vi "DiffDriveVoltageConstraint_getMinMaxAccel.vi"(8 "Velocity":dbl, 9 "Curvature":dbl, 10 "statePose":T5={"TRANSLATION"={"X"=0.0, "Y"=0.0}, "ROTATION"={"VALUE"=0.0, "COS"=1.0, "SIN"=0.0}} {"ROTATION"."SIN" format="%13.4f"; "ROTATION"."COS" format="%13.4f"; "ROTATION"."VALUE" format="%13.4f"; "TRANSLATION"."Y" format="%14.3f"; "TRANSLATION"."X" format="%14.3f"}, 11 "DIFF_DRIVE_VOLTAGE_CONSTRAINT":T1 {"SIMPLE_MOTOR_FF"."Ka" format="%13.4f"; "SIMPLE_MOTOR_FF"."Kv" format="%13.4f"; "SIMPLE_MOTOR_FF"."Ks" format="%13.4f"; "DIFF_DRIVE_KINEMATICS"."TrackWidth_Meters" format="%20.4f"; "Max Voltage" format="%20.4f"}) -> (3 "TRAJ_CONSTAINT_MIN_MAX":T4)   [LabVIEW 2019, in "Trajectory_Library.lvlib"]
doc: "Return the minimum and maximum allowed acceleration given the provided conditions.\n\nIt appears that this routine doesn't do anything. It returns default values.\n\nParameters:\n - DiffDriveVoltageConstraint - Constraint data structure\n - statePose - current traj state Pose\n - curvature - current traj curvature\n - maxVelocity - current traj max velocity\n\nReturns\n - TrajConstraint_Min_Max - Data structure with Min / Max acceleration."
uses:
  Trajectory_Library.lvlib
  TypeDef/POSE2D.ctl
  TypeDef/TRANSLATION2D.ctl
  TypeDef/ROTATION2D.ctl
  TypeDef/TRAJ_CONSTRAINT_MINMAX.ctl
  TypeDef/TRAJ_CONSTRAINT_DIIF_DRIVE_VOLTAGE.ctl
  TypeDef/DIFF_DRIVE_KINEMATICS.ctl
  TypeDef/SIMPLE_MOTOR_FF.ctl
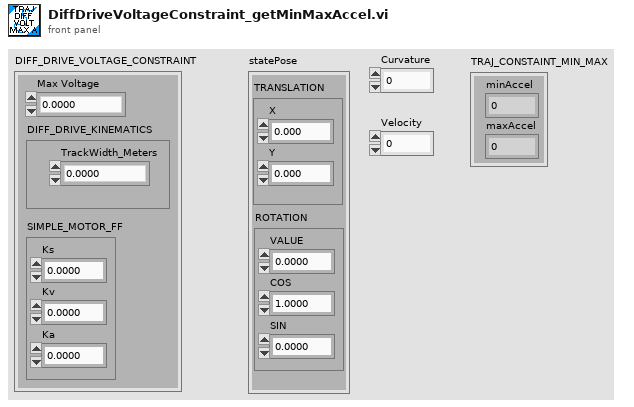
[diagram p1: front panel]
types:
  T1 = typedef "Trajectory_Library.lvlib/TRAJ_CONSTRAINT_DIIF_DRIVE_VOLTAGE.ctl" = cluster{"Max Voltage":dbl, "DIFF_DRIVE_KINEMATICS":T2, "SIMPLE_MOTOR_FF":T3}
  T2 = typedef "Trajectory_Library.lvlib/DIFF_DRIVE_KINEMATICS.ctl" = cluster{"TrackWidth_Meters":dbl}
  T3 = typedef "Trajectory_Library.lvlib/SIMPLE_MOTOR_FF.ctl" = cluster{"Ks":dbl, "Kv":dbl, "Ka":dbl}
  T4 = typedef "Trajectory_Library.lvlib/TRAJ_CONSTRAINT_MINMAX.ctl" = cluster{"minAccel":dbl, "maxAccel":dbl}
  T5 = typedef "Trajectory_Library.lvlib/POSE2D.ctl" = cluster{"TRANSLATION":T6, "ROTATION":T7}
  T6 = typedef "Trajectory_Library.lvlib/TRANSLATION2D.ctl" = cluster{"X":dbl, "Y":dbl}
  T7 = typedef "Trajectory_Library.lvlib/ROTATION2D.ctl" = cluster{"VALUE":dbl, "COS":dbl, "SIN":dbl}
  T8 = typedef "Trajectory_Library.lvlib/CHASSIS_SPEEDS.ctl" = cluster{"vX":dbl, "vY":dbl, "vOmega":dbl}
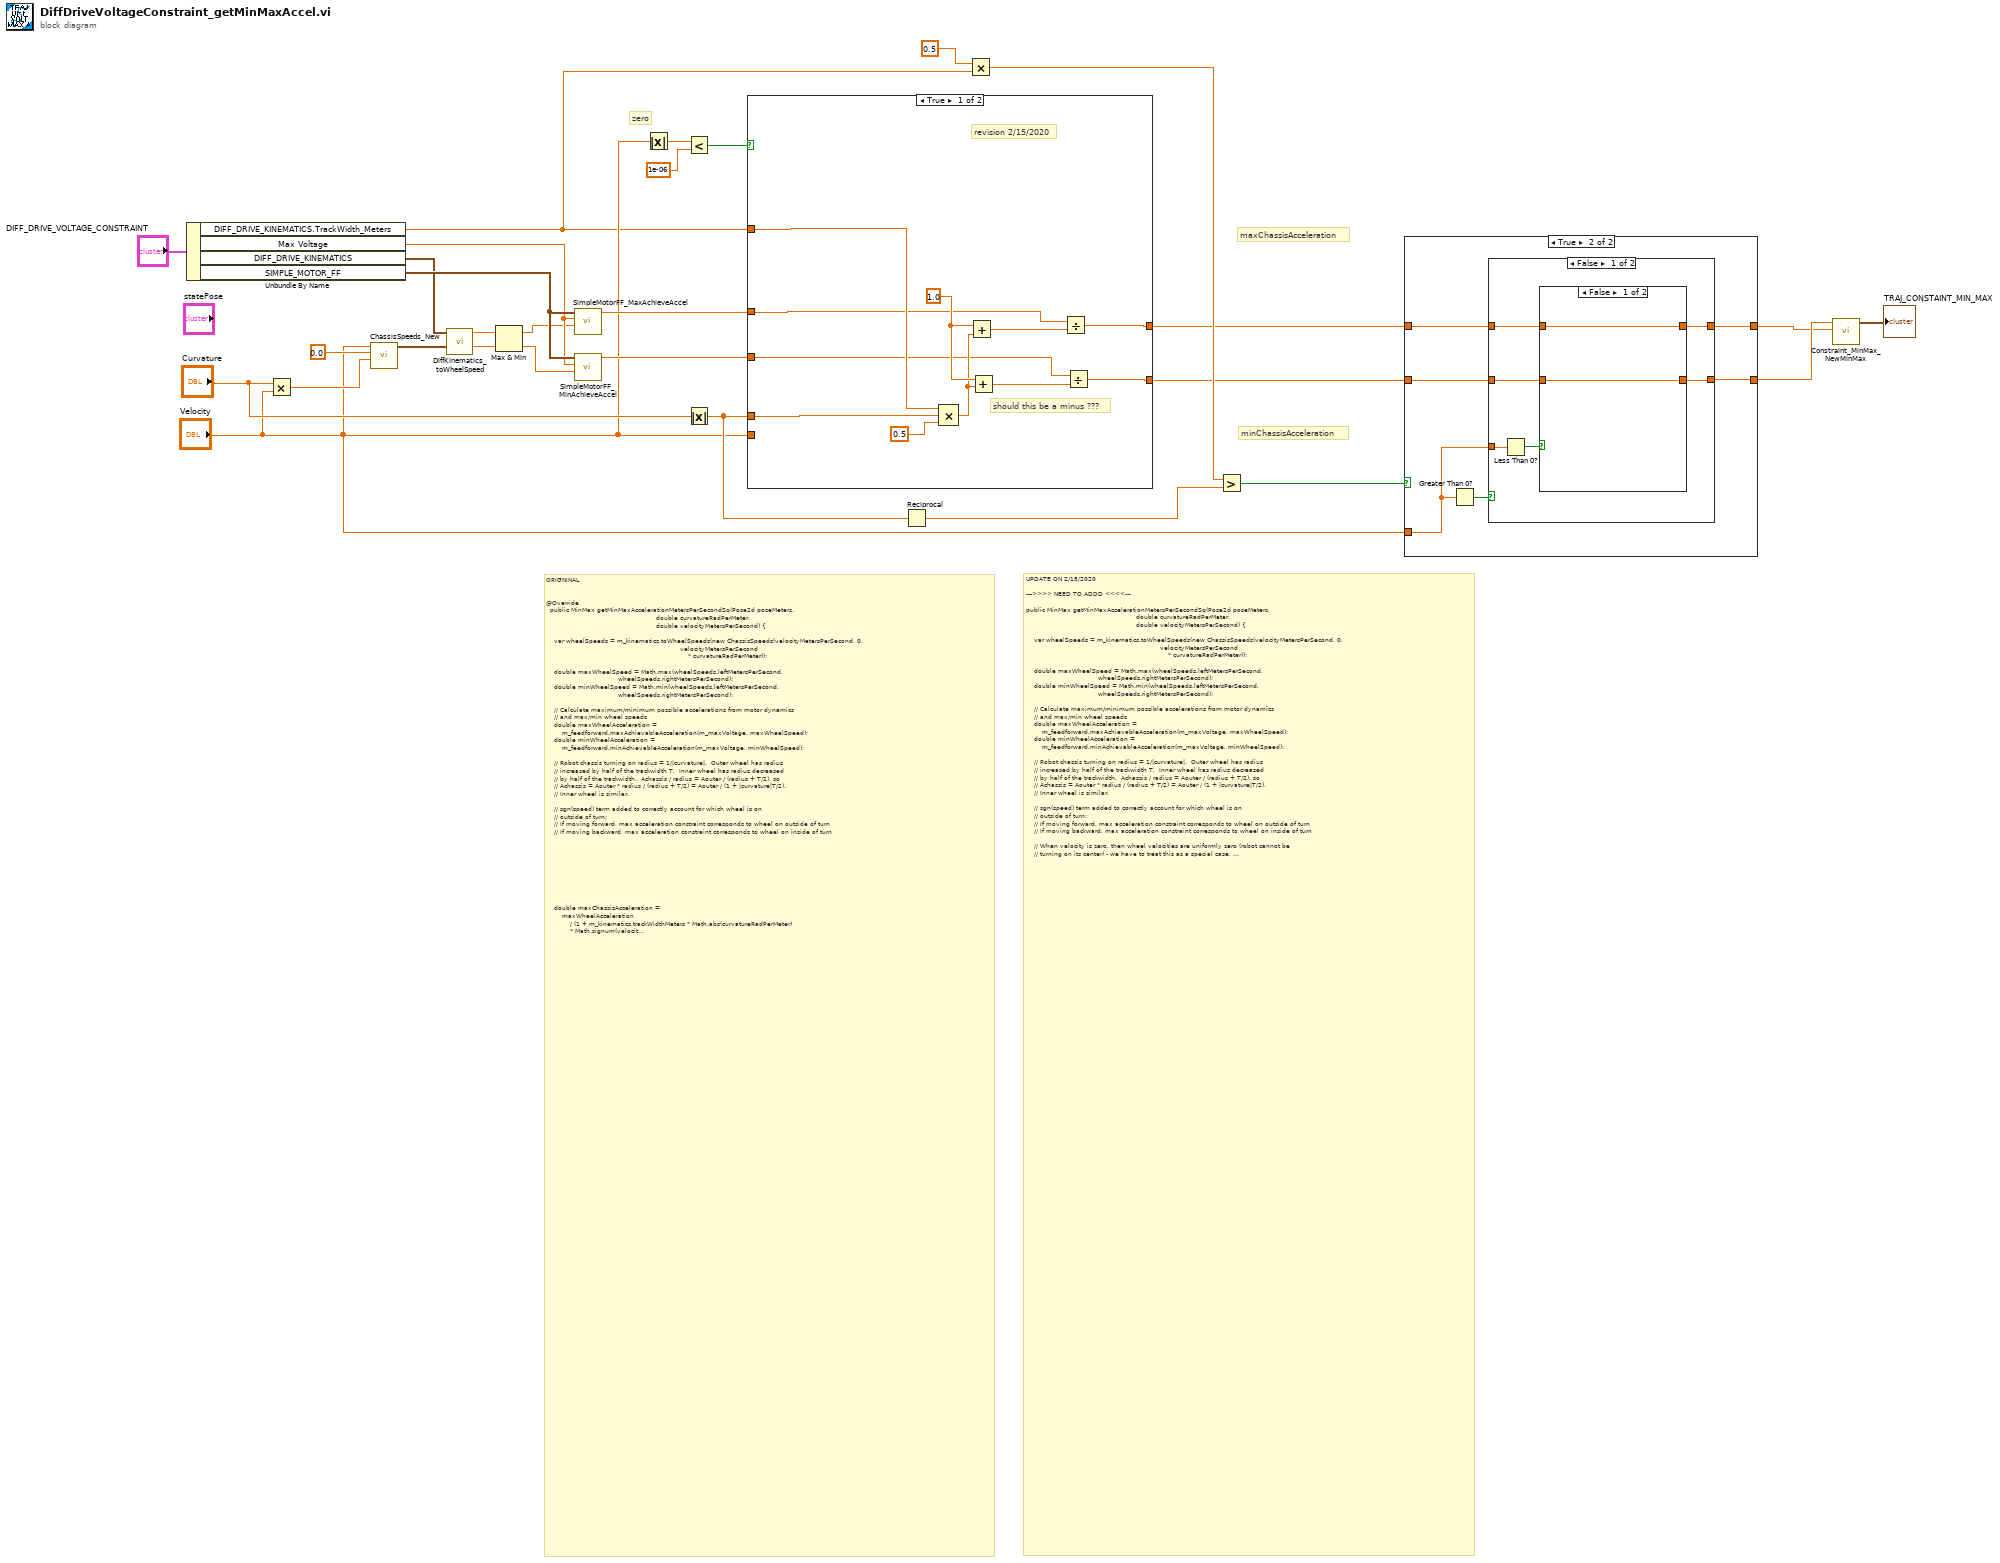
[diagram p0: block diagram]
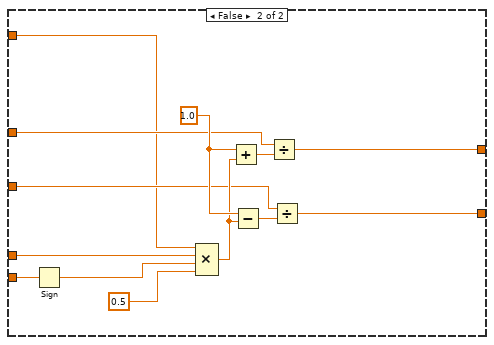
[diagram p2: hidden frame]
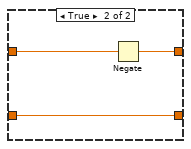
[diagram p4: hidden frame]
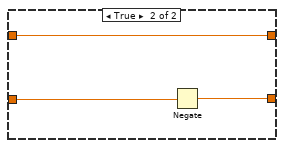
[diagram p5: hidden frame]
diagram:
  # "minChassisAcceleration"
  # "maxChassisAcceleration"
  # "zero"
  # "UPDATE ON 2/15/2020\n\n--->>>> NEED TO ADDD <<<<---\n\npublic MinMax getMinMaxAccelerationMetersPerSecondSq(Pose2d poseMeters,\n                                                       double curvatureRadPerMeter,\n                                                       double velocityMetersPerSecond) {\n\n    var wheelSpeeds = m_kinematics.toWheelSpeeds(new ChassisSpeeds(velocityMetersPerSecond, 0,\n                                                                   velocityMetersPerSecond\n                                                                       * curvatureRadPerMeter));\n\n    double maxWheelSpeed = Math.max(wheelSpeeds.leftMetersPerSecond,\n                                    wheelSpeeds.rightMetersPerSecond);\n    double minWheelSpeed = Math.min(wheelSpeeds.leftMetersPerSecond,\n                                    wheelSpeeds.rightMetersPerSecond);\n\n    // Calculate maximum/minimum possible accelerations from motor dynamics\n    // and max/min wheel speeds\n    double maxWheelAcceleration =\n        m_feedforward.maxAchievableAcceleration(m_maxVoltage, maxWheelSpeed);\n    double minWheelAcceleration =\n        m_feedforward.minAchievableAcceleration(m_maxVoltage, minWheelSpeed);\n\n    // Robot chassis turning on radius = 1/|curvature|.  Outer wheel has radius\n    // increased by half of the trackwidth T.  Inner wheel has radius decreased\n    // by half of the trackwidth.  Achassis / radius = Aouter / (radius + T/2), so\n    // Achassis = Aouter * radius / (radius + T/2) = Aouter / (1 + |curvature|T/2).\n    // Inner wheel is similar.\n\n    // sgn(speed) term added to correctly account for which wheel is on\n    // outside of turn:\n    // If moving forward, max acceleration constraint corresponds to wheel on outside of turn\n    // If moving backward, max acceleration constraint corresponds to wheel on inside of turn\n\n    // When velocity is zero, then wheel velocities are uniformly zero (robot cannot be\n    // turning on its center) - we have to treat this as a special case, as it breaks\n    // the signum function.  Both max and min acceleration are *reduced in magnitude*\n    // in this case.\n\n    double maxChassisAcceleration;\n    double minChassisAcceleration;\n\n    if (velocityMetersPerSecond == 0) {\n      maxChassisAcceleration =\n          maxWheelAcceleration\n              / (1 + m_kinematics.trackWidthMeters * Math.abs(curvatureRadPerMeter) / 2);\n      minChassisAcceleration =\n          minWheelAcceleration\n              / (1 + m_kinematics.trackWidthMeters * Math.abs(curvatureRadPerMeter) / 2);\n    } else {\n      maxChassisAcceleration =\n          maxWheelAcceleration\n              / (1 + m_kinematics.trackWidthMeters * Math.abs(curvatureRadPerMeter)\n              * Math.signum(velocityMetersPerSecond) / 2);\n      minChassisAcceleration =\n          minWheelAcceleration\n              / (1 - m_kinematics.trackWidthMeters * Math.abs(curvatureRadPerMeter)\n              * Math.signum(velocityMetersPerSecond) / 2);\n    }\n\n    // When turning about a point inside of the wheelbase (i.e. radius less than half\n    // the trackwidth), the inner wheel's direction changes, but the magnitude remains\n    // the same.  The formula above changes sign for the inner wheel when this happens.\n    // We can accurately account for this by simply negating the inner wheel.\n\n    if ((m_kinematics.trackWidthMeters / 2) > (1 / Math.abs(curvatureRadPerMeter))) {\n      if (velocityMetersPerSecond > 0) {\n        minChassisAcceleration = -minChassisAcceleration;\n      } else if (velocityMetersPerSecond < 0) {\n        maxChassisAcceleration = -maxChassisAcceleration;\n      }\n    }\n\n    return new MinMax(minChassisAcceleration, maxChassisAcceleration);\n  }\n}"
  # "ORIGNINAL\n\n\n@Override\n  public MinMax getMinMaxAccelerationMetersPerSecondSq(Pose2d poseMeters,\n                                                       double curvatureRadPerMeter,\n                                                       double velocityMetersPerSecond) {\n\n    var wheelSpeeds = m_kinematics.toWheelSpeeds(new ChassisSpeeds(velocityMetersPerSecond, 0,\n                                                                   velocityMetersPerSecond\n                                                                       * curvatureRadPerMeter));\n\n    double maxWheelSpeed = Math.max(wheelSpeeds.leftMetersPerSecond,\n                                    wheelSpeeds.rightMetersPerSecond);\n    double minWheelSpeed = Math.min(wheelSpeeds.leftMetersPerSecond,\n                                    wheelSpeeds.rightMetersPerSecond);\n\n    // Calculate maximum/minimum possible accelerations from motor dynamics\n    // and max/min wheel speeds\n    double maxWheelAcceleration =\n        m_feedforward.maxAchievableAcceleration(m_maxVoltage, maxWheelSpeed);\n    double minWheelAcceleration =\n        m_feedforward.minAchievableAcceleration(m_maxVoltage, minWheelSpeed);\n\n    // Robot chassis turning on radius = 1/|curvature|.  Outer wheel has radius\n    // increased by half of the trackwidth T.  Inner wheel has radius decreased\n    // by half of the trackwidth.  Achassis / radius = Aouter / (radius + T/2), so\n    // Achassis = Aouter * radius / (radius + T/2) = Aouter / (1 + |curvature|T/2).\n    // Inner wheel is similar.\n\n    // sgn(speed) term added to correctly account for which wheel is on\n    // outside of turn:\n    // If moving forward, max acceleration constraint corresponds to wheel on outside of turn\n    // If moving backward, max acceleration constraint corresponds to wheel on inside of turn\n\n\n\n\n\n\n\n\n\n    double maxChassisAcceleration =\n        maxWheelAcceleration\n            / (1 + m_kinematics.trackWidthMeters * Math.abs(curvatureRadPerMeter)\n            * Math.signum(velocityMetersPerSecond) / 2);\n    double minChassisAcceleration =\n        minWheelAcceleration\n            / (1 - m_kinematics.trackWidthMeters * Math.abs(curvatureRadPerMeter)\n            * Math.signum(velocityMetersPerSecond) / 2);\n\n\n\n\n\n\n\n\n\n\n\n\n\n\n    // Negate acceleration of wheel on inside of turn if center of turn is inside of wheelbase\n    if ((m_kinematics.trackWidthMeters / 2) > (1 / Math.abs(curvatureRadPerMeter))) {\n      if (velocityMetersPerSecond > 0) {\n        minChassisAcceleration = -minChassisAcceleration;\n      } else {\n        maxChassisAcceleration = -maxChassisAcceleration;\n      }\n    }\n\n    return new MinMax(minChassisAcceleration, maxChassisAcceleration);\n  }"
  n1 = Unbundle By Name("DIFF_DRIVE_VOLTAGE_CONSTRAINT") -> ("DIFF_DRIVE_KINEMATICS.TrackWidth_Meters"=w2:dbl, "Max Voltage"=w27:dbl, "DIFF_DRIVE_KINEMATICS"=w26:T2, "SIMPLE_MOTOR_FF"=w28:T3)
  n2 = Multiply(x="Curvature", y="Velocity") -> (x*y=w24:dbl)
  n3 = call "ChassisSpeeds_New.vi"("vAngular"=w24, "vY"=0.0 ("vAngular"), "vX"="Velocity") -> ("CHASSIS"=w23:T8)  [unwired: 8 in]
  n4 = call "DiffKinematics_toWheelSpeed.vi"("CHASSIS Speed"=w23, "DIFF_DRIVE_KINEMATICS"=w26) -> ("RightVelocity"=w22:dbl, "LeftVelocity"=w21:dbl)  [unwired: 8 in]
  n5 = Max & Min(x=w21, y=w22) -> (max(x,y)=w20:dbl, min(x,y)=w19:dbl)
  n6 = call "SimpleMotorFF_MaxAchieveAccel.vi"("Velocity"=w20, "MaxVoltage"=w27, "SIMPLE_MOTOR_FF"=w28) -> ("MaxAccel"=w17:dbl)  [unwired: 8 in]
  n7 = call "SimpleMotorFF_MinAchieveAccel.vi"("Velocity"=w19, "MaxVoltage"=w27, "SIMPLE_MOTOR_FF"=w28) -> ("MinAccel"=w16:dbl)  [unwired: 8 in]
  n8 = Absolute Value(x="Velocity") -> (abs(x)=w5:dbl)
  n9 = Less?(x=w5, y=1e-06) -> (x < y?=w1:bool)
  n10 = Absolute Value(x="Curvature") -> (abs(x)=w12:dbl)
  n11 = case shown="True" w1 {
    tunnel: w17 -> [w33 w47]
    tunnel: w16 -> [w32 w46]
    tunnel: w12 -> [w31 w45]
    tunnel: [w36 w44] -> w10
    tunnel: [w35 w43] -> w9
    tunnel: "Velocity" -> [_ w42]
    tunnel: w2 -> [w34 w41]
    frame True {
      w40 = 1.0 ("x")
      # "revision 2/15/2020"
      # "should this be a minus ???"
      n12 = Compound Arithmetic op=MULTIPLY(w34, w31, 0.5 ("value")) -> (w39:dbl)
      n13 = Add(x=w40, y=w39) -> (x+y=w38:dbl)
      n14 = Add(x=w40, y=w39) -> (x+y=w37:dbl)
      n15 = Divide(x=w33, y=w38) -> (x/y=w36:dbl)
      n16 = Divide(x=w32, y=w37) -> (x/y=w35:dbl)
    }
    frame False {
      w51 = 1.0 ("x")
      n17 = Sign(1:w42) -> (0:w53:dbl)
      n18 = Compound Arithmetic op=MULTIPLY(w41, w45, w53, 0.5 ("value")) -> (w50:dbl)
      n19 = Add(x=w51, y=w50) -> (x+y=w49:dbl)
      n20 = Subtract(x=w51, y=w50) -> (x-y=w48:dbl)
      n21 = Divide(x=w47, y=w49) -> (x/y=w44:dbl)
      n22 = Divide(x=w46, y=w48) -> (x/y=w43:dbl)
    }
  }
  n23 = Reciprocal(x=w12) -> (1/x=w11:dbl)
  n24 = Multiply(x=0.5, y=w2) -> (x*y=w13:dbl)
  n25 = Greater?(x=w13, y=w11) -> (0:w14:bool)
  n26 = case shown="True" w14 {
    tunnel: w10 -> [w54 w58]
    tunnel: w9 -> [w55 w60]
    tunnel: [w55 w59] -> w8
    tunnel: [w54 w57] -> w7
    tunnel: "Velocity" -> [_ w56]
    frame False {
    }
    frame True {
      n27 = Greater Than 0?(x=w56) -> (x > 0?=w61:bool)
      n28 = case shown="False" w61 {
        tunnel: w60 -> [w64 w75]
        tunnel: [w63 w74] -> w59
        tunnel: w58 -> [w67 w73]
        tunnel: [w66 w73] -> w57
        tunnel: w56 -> [w65 _]
        frame False {
          n29 = Less Than 0?(x=w65) -> (x < 0?=w62:bool)
          n30 = case shown="False" w62 {
            tunnel: w67 -> [w69 w72]
            tunnel: [w69 w71] -> w66
            tunnel: w64 -> [w68 w70]
            tunnel: [w68 w70] -> w63
            frame False {
            }
            frame True {
              n31 = Negate(x=w72) -> (-x=w71:dbl)
            }
          }
        }
        frame True {
          n32 = Negate(x=w75) -> (-x=w74:dbl)
        }
      }
    }
  }
  n33 = call "Constraint_MinMax_NewMinMax.vi"("Max"=w7, "Min"=w8) -> ("TRAJ_CONSTAINT_MIN_MAX"=→"TRAJ_CONSTAINT_MIN_MAX":T4)  [unwired: 9 in]
